vi "电源管理UI.vi"() -> ()   [LabVIEW 2016, in "PLC.lvlib"]
uses:
  PLC.lvlib
  <vilib>/Utility/miscctls.llb/LVPointTypeDef.ctl
  API/CodCr/CodCr.lvlib
  <vilib>/ptbypt/NI_PtbyPt.lvlib
panel:
  out "总氮空闲时间":dbl caption="空闲时间:"
  in  "总氮电源":bool
  out "CODCr空闲时间":dbl caption="空闲时间:"
  out "总磷空闲时间":dbl caption="空闲时间:"
  out "营养盐空闲时间":dbl caption="空闲时间:"
  out "CODMn空闲时间":dbl caption="空闲时间:"
  out "多参数空闲时间":dbl caption="空闲时间:"
  in  "CODCr电源":bool
  in  "总磷电源":bool
  in  "氨氮电源":bool
  in  "CODMn电源":bool
  in  "多参数电源":bool
  # "说明：\n系统模式处于维护模式时，仪器电源自动打开；\n系统模式处于常规模式/质控模式/应急模式下，周期启动时，仪器电源打开，仪器空闲超过3600秒自动断电；"
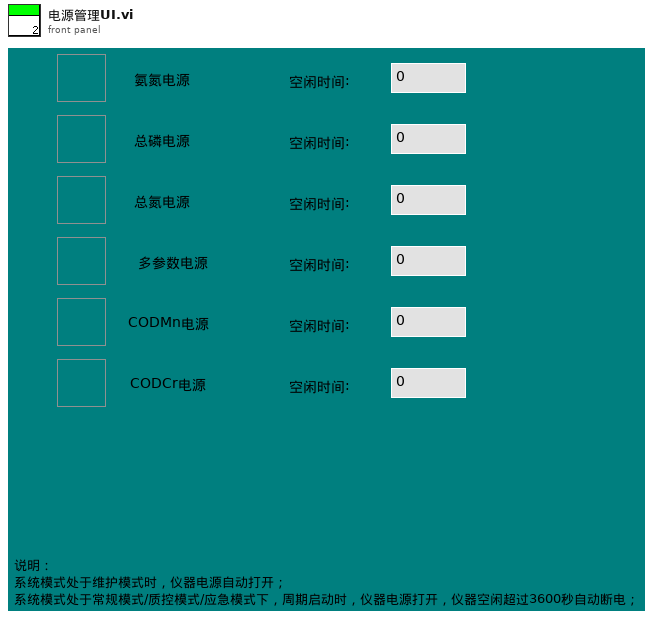
[diagram p1: front panel]
types:
  T1 = typedef "LVPointTypeDef.ctl" = cluster{"Horizontal":i16, "Vertical":i16}
  T2 = cluster{"测量量程":dbl, "测量精度":dbl, "测量间隔":dbl, "消解温度":dbl, "消解时长":dbl, "空白校准时间":timestamp, "曲线截距":dbl, "曲线斜率":dbl, "测量检出限":dbl, "测量信号值":dbl, "线性相关系数":dbl, "二次多项式系数":dbl, "标样校准时间":timestamp}
  T3 = cluster{"测量精度":u16, "消解温度":u16, "消解时长":u16, "量程下限":sgl, "量程上限":sgl, "曲线斜率K":sgl, "曲线斜率B":sgl, "标定日期":timestamp, "标液1浓度":sgl, "标液1测量过程值":sgl, "标液2浓度":sgl, "标液2测量过程值":sgl, "标液3浓度":sgl, "标液3测量过程值":sgl, "标液4浓度":sgl, "标液4测量过程值":sgl, "标液5浓度":sgl, "标液5测量过程值":sgl, "线性相关系数":sgl, "试剂余量":u32, "测量滴定值或吸光度":sgl, "空白校准时间":timestamp, "标样校准时间":timestamp, "检出限值":sgl, "校准系数":sgl, "设备系列号":string}
  T4 = enum16{"空闲", "水样测试", "标样核查", "零点核查", "跨度核查", "空白测试", "平行样测试", "加标回收", "空白校准", "标样校准", "初始化（清洗）"}
  T5 = cluster{"R0":i16, "R1":i16, "R2":i16, "R3":i16, "R4":i16, "R5":i16, "R6":i16, "R7":i16, "R8":i16, "R9":i16, "R10":i16, "R11":i16, "R12":i16, "R13":i16, "R14":i16, "R15":i16, "R16":i16, "R17":i16, "R18":i16, "R19":i16, "R20":i16, "R21":i16, "R22":i16, "R23":i16, "R24":i16, "R25":i16, "R26":i16, "R27":i16, "R28":i16, "R29":i16, "R30":i16, "R31":i16, "R32":i16, "R33":i16, "R34":i16, "R35":i16, "R36":i16, "R37":i16, "R38":i16, "R39":i16, "R40":i16, "R41":i16, "R42":i16, "R43":i16, "R44":i16, "R45":i16, "R46":i16, "R47":i16, "R48":i16, "R49":i16, "R50":i16, "R51":i16, "R52":i16, "R53":i16, "R54":i16, "R55":i16, "R56":i16}
  T6 = cluster{"系统时间":timestamp, "工作状态":enum16{"空闲", "水样测试", "标样核查", "零点核查", "跨度核查", "空白测试", "平行样测试", "加标回收", "空白校准", "标样校准", "初始化（清洗）"}, "测量模式":enum16{"待机", "连续模式", "周期模式", "定点模式", "受控模式", "手动模式"}, "告警代码":enum16{"无告警", "缺试剂告警", "缺水样告警", "缺蒸馏水告警", "缺标液告警", "仪表漏液告警", "标定异常告警", "超量程告警", "加热异常", "低试剂预警", "超上限告警", "超下限告警", "仪表内部其他异常", "滴定异常告警", "电极异常告警", "量程切换告警", "参数设置告警", "PH电极电位异常", "电导率电极异常", "浊度光度异常", "溶解氧电极异常", "溶解氧光强异常", "温度异常告警", "PH异常告警", "溶解氧异常告警", "电导率异常告警", "浊度异常告警", "叶绿素异常告警", "藻密度异常告警", "蓝绿藻异常告警", "ORP异常告警", "氨氮异常告警", "清洁刷异常告警", "SD卡异常告警", "蓝牙异常告警", "Wifi异常告警", "流程异常告警"}, "故障代码":enum16{"无故障", "电机故障", "温度故障", "通讯故障", "滴定故障"}, "日志代码":u16, "软件版本":u16, "F0":sgl, "F1":sgl, "F2":sgl, "F3":sgl, "T":sgl, "H":sgl, "id":u16, "flowid":u16, "量程":u16, "总磷控温温度1":sgl, "营养盐控温温度2":sgl, "ADC":sgl}
  T7 = cluster{"系统时间":timestamp, "工作状态":u16, "测量模式":u16, "告警代码":enum16{"无告警", "缺试剂告警", "缺水样告警", "缺蒸馏水告警", "缺标液告警", "仪表漏液告警", "标定异常告警", "超量程告警", "加热异常", "低试剂预警", "超上限告警", "超下限告警", "仪表内部其他异常", "滴定异常告警", "电极异常告警", "量程切换告警", "参数设置告警", "PH电极电位异常", "电导率电极异常", "浊度光度异常", "溶解氧电极异常", "溶解氧光强异常", "温度异常告警", "PH异常告警", "溶解氧异常告警", "电导率异常告警", "浊度异常告警", "叶绿素异常告警", "藻密度异常告警", "蓝绿藻异常告警", "ORP异常告警", "氨氮异常告警", "清洁刷异常告警", "SD卡异常告警", "蓝牙异常告警", "Wifi异常告警", "流程异常告警"}, "故障代码":enum16{"无故障", "电机故障", "温度故障", "通讯故障", "滴定故障"}, "日志代码":u16, "软件版本":string}
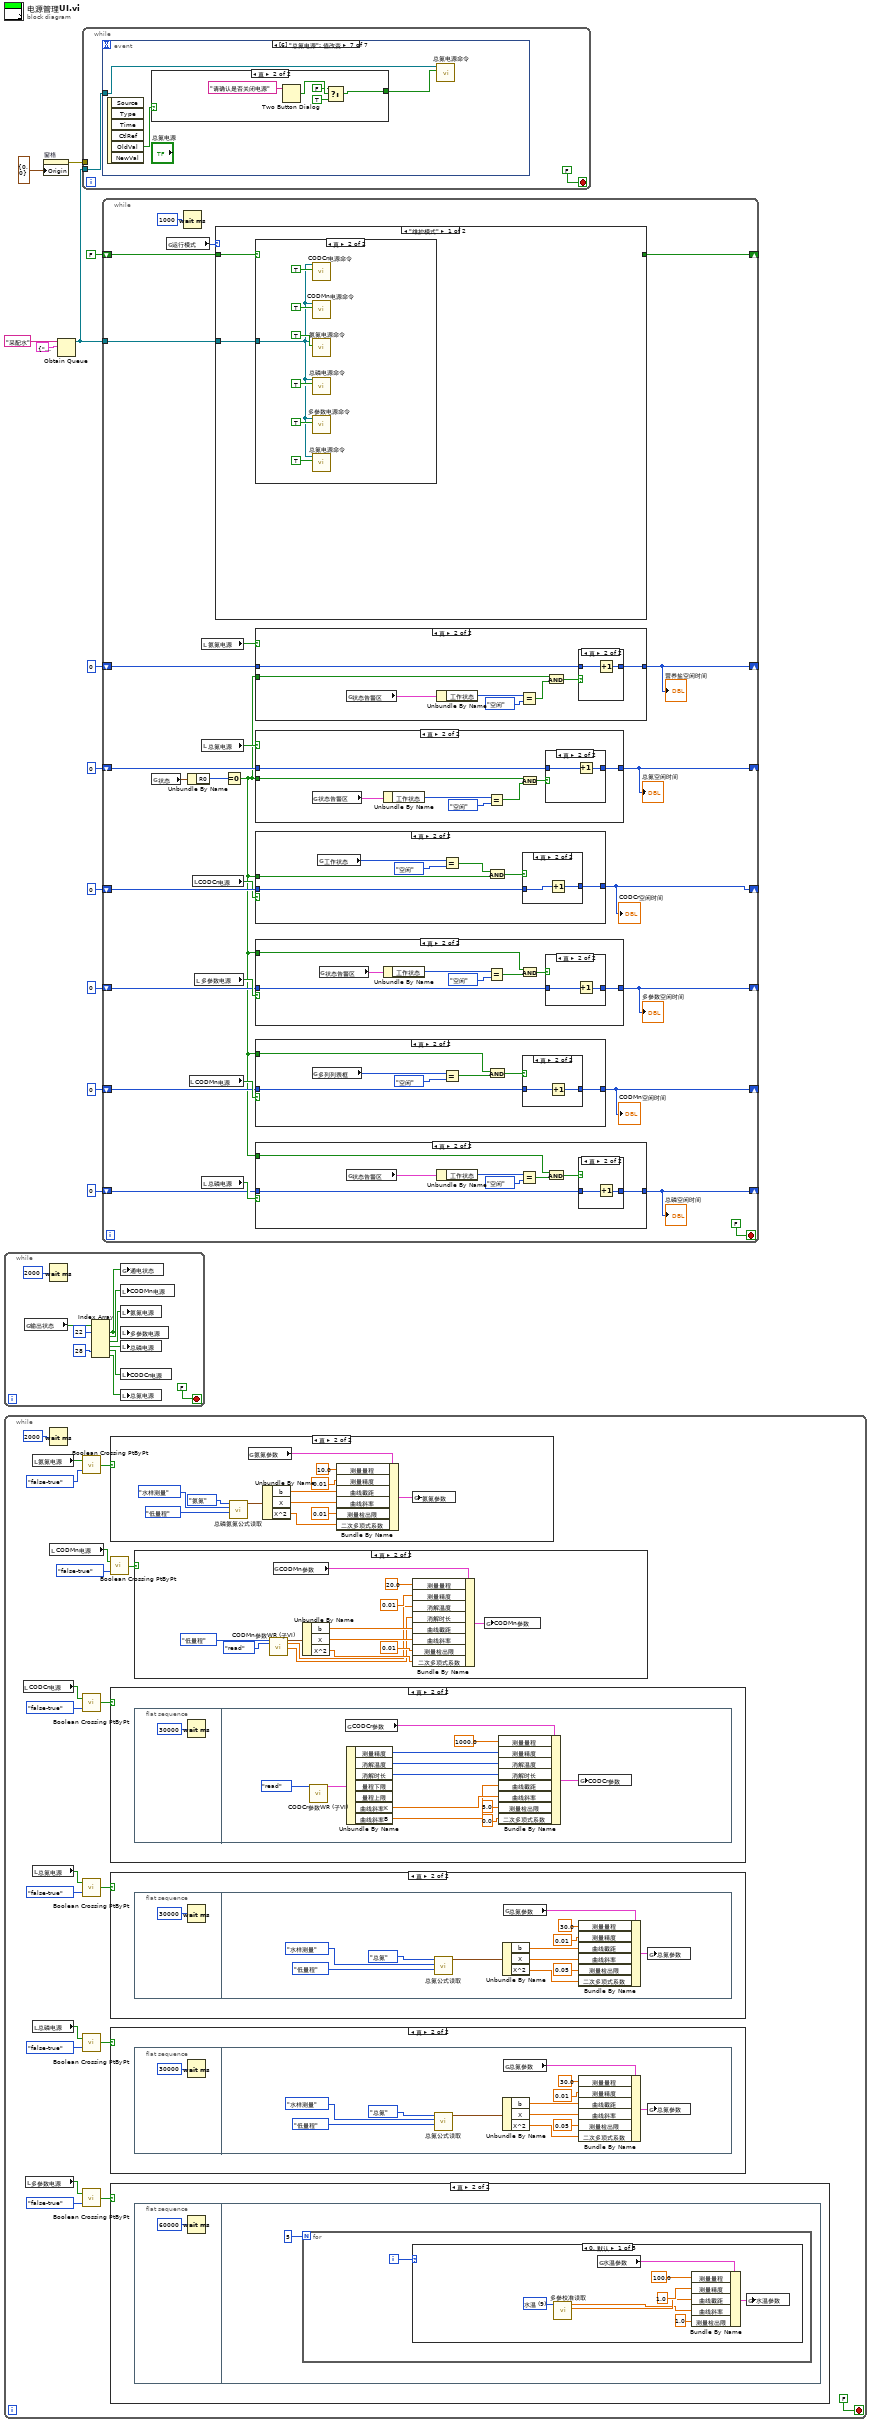
[diagram p0: block diagram]
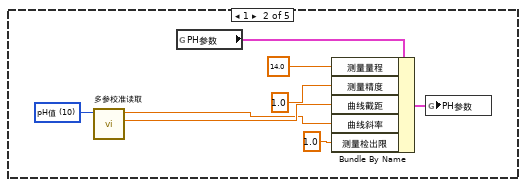
[diagram p8: hidden frame]
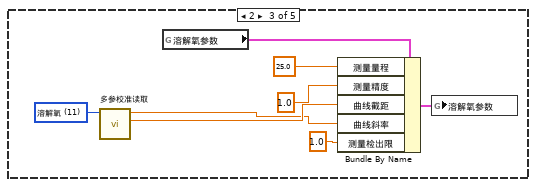
[diagram p9: hidden frame]
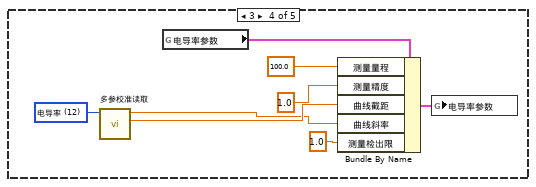
[diagram p10: hidden frame]
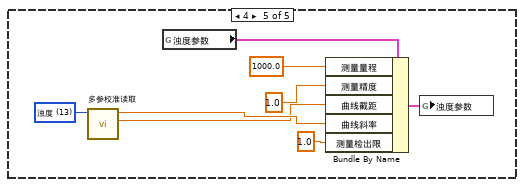
[diagram p11: hidden frame]
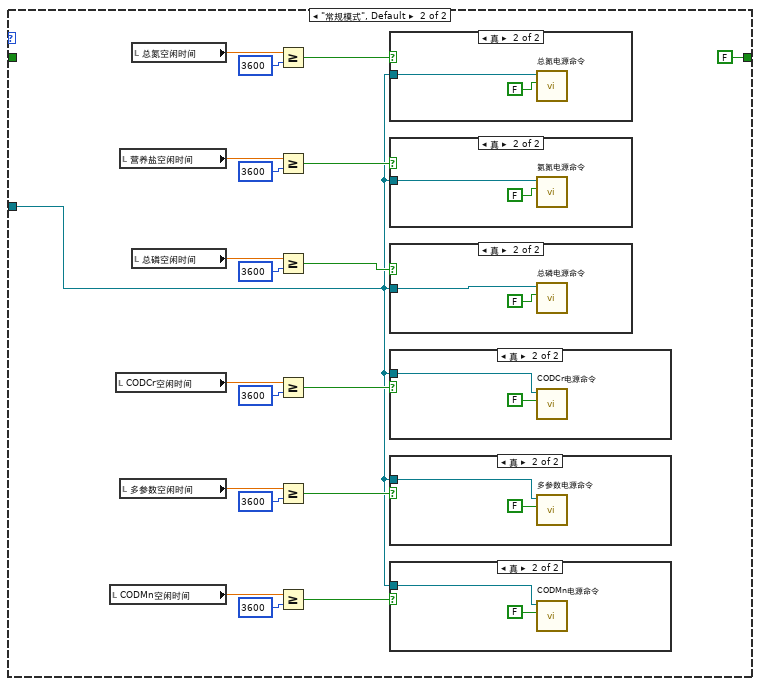
[diagram p15: hidden frame]
diagram:
  n1 = while {
    stop <- FALSE stop-if-true
    n2 = global read "采配水全局变量.vi" "输出状态"() -> (w21:bool[])
    n3 = Wait (ms)(milliseconds to wait=u32 2000 ("等待时间（毫秒）")) -> ()  [unwired: 1 out]
    n4 = Index Array(array=w21, index #1=22 ("索引"), index #5=28 ("索引")) -> (element #1=w16:bool, element #2=w19:bool, element #3=w18:bool, element #4=w17:bool, element #5=w14:bool, element #6=w13:bool)  [unwired: 4 in]
    n5 = global write "多参数全局变量.vi" "通电状态"(w16) -> ()
    n6 = local write "CODMn电源"(w19) -> ()
    n7 = local write "氨氮电源"(w18) -> ()
    n8 = local write "多参数电源"(w16) -> ()
    n9 = local write "总磷电源"(w17) -> ()
    n10 = local write "CODCr电源"(w14) -> ()
    n11 = local write "总氮电源"(w13) -> ()
  }
  n12 = while {
    stop <- FALSE stop-if-true
    n13 = local read "CODCr电源"() -> (w25:bool)
    n14 = local read "多参数电源"() -> (w41:bool)
    n15 = local read "氨氮电源"() -> (w34:bool)
    n16 = local read "总氮电源"() -> (w28:bool)
    n17 = local read "总磷电源"() -> (w31:bool)
    n18 = Wait (ms)(milliseconds to wait=u32 2000 ("等待时间（毫秒）")) -> ()  [unwired: 1 out]
    n19 = local read "CODMn电源"() -> (w37:bool)
    n20 = call <vilib>:"Boolean Crossing PtByPt.vi"("direction"=enum16{"either", "false-true", "true-false"}."false-true", "input"=w34) -> ("crossing"=w33:bool)  [unwired: 1 in]
    n21 = call <vilib>:"Boolean Crossing PtByPt.vi"("direction"=enum16{"either", "false-true", "true-false"}."false-true", "input"=w25) -> ("crossing"=w24:bool)  [unwired: 1 in]
    n22 = call <vilib>:"Boolean Crossing PtByPt.vi"("direction"=enum16{"either", "false-true", "true-false"}."false-true", "input"=w28) -> ("crossing"=w29:bool)  [unwired: 1 in]
    n23 = call <vilib>:"Boolean Crossing PtByPt.vi"("direction"=enum16{"either", "false-true", "true-false"}."false-true", "input"=w31) -> ("crossing"=w30:bool)  [unwired: 1 in]
    n24 = call <vilib>:"Boolean Crossing PtByPt.vi"("direction"=enum16{"either", "false-true", "true-false"}."false-true", "input"=w41) -> ("crossing"=w39:bool)  [unwired: 1 in]
    n25 = case shown="真" w33 {
      frame False {
      }
      frame True {
        n26 = call "总磷氨氮公式读取.vi"("量程"=enum16{"低量程", "高量程"}."低量程", "测量模式"=enum16{"水样测量", "空白核查", "跨度核查", "标样核查", "加标回收"}."水样测量", "测量参数"=enum16{"氨氮", "总磷"}."氨氮") -> ("公式"=w83:cluster{"X^2":dbl, "X":dbl, "b":dbl})  [unwired: 7 in, 1 out]
        n27 = global read "在线监测仪器仪表参数.vi" "氨氮参数"() -> (w87:T2)
        n28 = Unbundle By Name(w83) -> ("b"=w91:dbl, "X"=w92:dbl, "X^2"=w93:dbl)
        n29 = Bundle By Name(cluster=w87, "测量量程"=10.0, "测量精度"=0.01, "曲线截距"=w91, "曲线斜率"=w92, "测量检出限"=0.01, "二次多项式系数"=w93) -> (w88:T2)
        n30 = global write "在线监测仪器仪表参数.vi" "氨氮参数"(w88) -> ()
      }
    }
    n31 = call <vilib>:"Boolean Crossing PtByPt.vi"("direction"=enum16{"either", "false-true", "true-false"}."false-true", "input"=w37) -> ("crossing"=w36:bool)  [unwired: 1 in]
    n32 = case shown="真" w24 {
      frame False {
      }
      frame True {
        n33 = flat-sequence {
          frame #0 {
            n34 = Wait (ms)(milliseconds to wait=u32 30000 ("等待时间（毫秒）")) -> ()  [unwired: 1 out]
          }
          frame #1 {
            n35 = call "CODCr参数WR (子VI) .vi"("STEP"=enum16{"read", "writekb", "写入消解温度时间"}."read") -> ("关键参数区"=w46:T3)  [unwired: 17 in, 1 out]
            n36 = global read "在线监测仪器仪表参数.vi" "CODCr参数"() -> (w54:T2)
            n37 = Unbundle By Name(w46) -> ("测量精度"=w53:u16, "消解温度"=w47:u16, "消解时长"=w48:u16, "曲线斜率K"=w50:sgl, "曲线斜率B"=w49:sgl)  [unwired: 2 out]
            n38 = Bundle By Name(cluster=w54, "测量量程"=1000.0, "测量精度"=w53, "消解温度"=w47, "消解时长"=w48, "曲线截距"=w49, "曲线斜率"=w50, "测量检出限"=5.0, "二次多项式系数"=0.0) -> (w55:T2)
            n39 = global write "在线监测仪器仪表参数.vi" "CODCr参数"(w55) -> ()
          }
        }
      }
    }
    n40 = case shown="真" w29 {
      frame False {
      }
      frame True {
        n41 = flat-sequence {
          frame #0 {
            n42 = Wait (ms)(milliseconds to wait=u32 30000 ("等待时间（毫秒）")) -> ()  [unwired: 1 out]
          }
          frame #1 {
            n43 = call "总氮公式读取.vi"("量程"=enum16{"低量程", "高量程"}."低量程", "测量模式"=enum16{"水样测量", "空白核查", "跨度核查", "标样核查", "加标回收"}."水样测量", "测量参数"=enum16{"总磷", "总氮"}."总氮") -> ("公式"=w58:cluster{"X^2":dbl, "X":dbl, "b":dbl})  [unwired: 7 in, 1 out]
            n44 = Unbundle By Name(w58) -> ("b"=w67:dbl, "X"=w68:dbl, "X^2"=w69:dbl)
            n45 = global read "在线监测仪器仪表参数.vi" "总氮参数"() -> (w66:T2)
            n46 = Bundle By Name(cluster=w66, "测量量程"=30.0, "测量精度"=0.01, "曲线截距"=w67, "曲线斜率"=w68, "测量检出限"=0.05, "二次多项式系数"=w69) -> (w65:T2)
            n47 = global write "在线监测仪器仪表参数.vi" "总氮参数"(w65) -> ()
          }
        }
      }
    }
    n48 = case shown="真" w30 {
      frame False {
      }
      frame True {
        n49 = flat-sequence {
          frame #0 {
            n50 = Wait (ms)(milliseconds to wait=u32 30000 ("等待时间（毫秒）")) -> ()  [unwired: 1 out]
          }
          frame #1 {
            n51 = call "总氮公式读取.vi"("量程"=enum16{"低量程", "高量程"}."低量程", "测量模式"=enum16{"水样测量", "空白核查", "跨度核查", "标样核查", "加标回收"}."水样测量", "测量参数"=enum16{"总磷", "总氮"}."总氮") -> ("公式"=w71:cluster{"X^2":dbl, "X":dbl, "b":dbl})  [unwired: 7 in, 1 out]
            n52 = Unbundle By Name(w71) -> ("b"=w80:dbl, "X"=w81:dbl, "X^2"=w82:dbl)
            n53 = global read "在线监测仪器仪表参数.vi" "总氮参数"() -> (w79:T2)
            n54 = Bundle By Name(cluster=w79, "测量量程"=30.0, "测量精度"=0.01, "曲线截距"=w80, "曲线斜率"=w81, "测量检出限"=0.05, "二次多项式系数"=w82) -> (w78:T2)
            n55 = global write "在线监测仪器仪表参数.vi" "总氮参数"(w78) -> ()
          }
        }
      }
    }
    n56 = case shown="真" w39 {
      frame False {
      }
      frame True {
        n57 = flat-sequence {
          frame #0 {
            n58 = Wait (ms)(milliseconds to wait=u32 60000 ("等待时间（毫秒）")) -> ()  [unwired: 1 out]
          }
          frame #1 {
            n59 = for {
              N: 5 -> [_]
              i -> [w110]
              n60 = case shown="0, 默认" w110 {
                frame 0, Default {
                  w113 = u16 9 items=["氨氮"=3, "水温"=9, "pH值"=10, "溶解氧"=11, "电导率"=12, "浊度"=13, "叶绿素a"=14, "藻密度"=15, "蓝绿藻"=16, "氧化还原电位"=17, "溶解氧%"=18, "盐度"=19] ("站号")
                  n61 = call "多参校准读取.vi"("站号"=w113) -> ("B"=w112:dbl, "K"=w111:dbl)  [unwired: 8 in, 1 out]
                  n62 = global read "在线监测仪器仪表参数.vi" "水温参数"() -> (w115:T2)
                  n63 = Bundle By Name(cluster=w115, "测量量程"=100.0, "测量精度"=1.0, "曲线截距"=w112, "曲线斜率"=w111, "测量检出限"=1.0) -> (w116:T2)
                  n64 = global write "在线监测仪器仪表参数.vi" "水温参数"(w116) -> ()
                }
                frame 1 {
                  w121 = u16 10 items=["氨氮"=3, "水温"=9, "pH值"=10, "溶解氧"=11, "电导率"=12, "浊度"=13, "叶绿素a"=14, "藻密度"=15, "蓝绿藻"=16, "氧化还原电位"=17, "溶解氧%"=18, "盐度"=19] ("站号")
                  n65 = call "多参校准读取.vi"("站号"=w121) -> ("B"=w120:dbl, "K"=w119:dbl)  [unwired: 8 in, 1 out]
                  n66 = global read "在线监测仪器仪表参数.vi" "PH参数"() -> (w123:T2)
                  n67 = Bundle By Name(cluster=w123, "测量量程"=14.0, "测量精度"=1.0, "曲线截距"=w120, "曲线斜率"=w119, "测量检出限"=1.0) -> (w124:T2)
                  n68 = global write "在线监测仪器仪表参数.vi" "PH参数"(w124) -> ()
                }
                frame 2 {
                  w129 = u16 11 items=["氨氮"=3, "水温"=9, "pH值"=10, "溶解氧"=11, "电导率"=12, "浊度"=13, "叶绿素a"=14, "藻密度"=15, "蓝绿藻"=16, "氧化还原电位"=17, "溶解氧%"=18, "盐度"=19] ("站号")
                  n69 = call "多参校准读取.vi"("站号"=w129) -> ("B"=w128:dbl, "K"=w127:dbl)  [unwired: 8 in, 1 out]
                  n70 = global read "在线监测仪器仪表参数.vi" "溶解氧参数"() -> (w131:T2)
                  n71 = Bundle By Name(cluster=w131, "测量量程"=25.0, "测量精度"=1.0, "曲线截距"=w128, "曲线斜率"=w127, "测量检出限"=1.0) -> (w132:T2)
                  n72 = global write "在线监测仪器仪表参数.vi" "溶解氧参数"(w132) -> ()
                }
                frame 3 {
                  w137 = u16 12 items=["氨氮"=3, "水温"=9, "pH值"=10, "溶解氧"=11, "电导率"=12, "浊度"=13, "叶绿素a"=14, "藻密度"=15, "蓝绿藻"=16, "氧化还原电位"=17, "溶解氧%"=18, "盐度"=19] ("站号")
                  n73 = call "多参校准读取.vi"("站号"=w137) -> ("B"=w136:dbl, "K"=w135:dbl)  [unwired: 8 in, 1 out]
                  n74 = global read "在线监测仪器仪表参数.vi" "电导率参数"() -> (w139:T2)
                  n75 = Bundle By Name(cluster=w139, "测量量程"=100.0, "测量精度"=1.0, "曲线截距"=w136, "曲线斜率"=w135, "测量检出限"=1.0) -> (w140:T2)
                  n76 = global write "在线监测仪器仪表参数.vi" "电导率参数"(w140) -> ()
                }
                frame 4 {
                  w145 = u16 13 items=["氨氮"=3, "水温"=9, "pH值"=10, "溶解氧"=11, "电导率"=12, "浊度"=13, "叶绿素a"=14, "藻密度"=15, "蓝绿藻"=16, "氧化还原电位"=17, "溶解氧%"=18, "盐度"=19] ("站号")
                  n77 = call "多参校准读取.vi"("站号"=w145) -> ("B"=w143:dbl, "K"=w144:dbl)  [unwired: 8 in, 1 out]
                  n78 = global read "在线监测仪器仪表参数.vi" "浊度参数"() -> (w147:T2)
                  n79 = Bundle By Name(cluster=w147, "测量量程"=1000.0, "测量精度"=1.0, "曲线截距"=w143, "曲线斜率"=w144, "测量检出限"=1.0) -> (w148:T2)
                  n80 = global write "在线监测仪器仪表参数.vi" "浊度参数"(w148) -> ()
                }
              }
            }
          }
        }
      }
    }
    n81 = case shown="真" w36 {
      frame False {
      }
      frame True {
        n82 = call "CODMn参数WR (子VI).vi"("量程选择"=enum16{"低量程", "高量程"}."低量程", "STEP"=enum16{"read", "writekb", "写入消解温度时间"}."read") -> ("方程系数"=w99:cluster{"X^2":dbl, "X":dbl, "b":dbl}, "消解温度"=w98:dbl, "恒温时间"=w97:dbl)  [unwired: 14 in, 1 out]
        n83 = global read "在线监测仪器仪表参数.vi" "CODMn参数"() -> (w100:T2)
        n84 = Unbundle By Name(w99) -> ("b"=w105:dbl, "X"=w106:dbl, "X^2"=w107:dbl)
        n85 = Bundle By Name(cluster=w100, "测量量程"=20.0, "测量精度"=0.01, "消解温度"=w98, "消解时长"=w97, "曲线截距"=w105, "曲线斜率"=w106, "测量检出限"=0.01, "二次多项式系数"=w107) -> (w101:T2)
        n86 = global write "在线监测仪器仪表参数.vi" "CODMn参数"(w101) -> ()
      }
    }
  }
  n87 = property on="窗格" class="Pane"("Origin"=T1 {"Horizontal"=0, "Vertical"=0} ("原点")) -> (error out=w9:errorcluster)  [unwired: 2 in, 1 out]
  n88 = Obtain Queue(name (unnamed)="采配水" ("名称（未命名）"), element data type=cluster{"命令":string, "数据":variant} {"命令"="", "数据"=variant}) -> (queue out=w8:refnum<queue>)  [unwired: 3 in, 2 out]
  n89 = while {
    tunnel: w8 -> [w151]
    tunnel: w9 -> [_]
    stop <- FALSE stop-if-true
    n90 = event shown="[6] \"总氮电源\": 值改变" {
      selector: _ -> [_ _ _ _ _ _ _]
      dyn-events: _ -> [_ _ _ _ _ _ _]
      timeout: _ -> [_ _ _ _ _ _ _]
      tunnel: w151 -> [_ w155 w164 w173 w182 w191 w200]
      event Timeout {
        n91 = event-data() -> ()  [unwired: 1 in, 3 out]
      }
      event "多参数电源": Value Change {
        n92 = event-data() -> ("OldVal"=w154:bool)  [unwired: 1 in, 5 out]
        n93 = case shown="真" w154 {
          tunnel: [TRUE ("T button?") w157] -> w153
          frame False {
          }
          frame True {
            n94 = Two Button Dialog(message="请确认是否关闭电源" ("消息")) -> (T button?=w160:bool)  [unwired: 2 in]
            n95 = Select(t=FALSE, s=w160, f=TRUE ("T button?")) -> (s? t:f=w157:bool)
          }
        }
        n96 = call "多参数电源命令.vi"("通电/断电"=w153, "队列"=w155) -> ()  [unwired: 9 in, 1 out]
      }
      event "CODMn电源": Value Change {
        n97 = event-data() -> ("OldVal"=w163:bool)  [unwired: 1 in, 5 out]
        n98 = case shown="真" w163 {
          tunnel: [TRUE ("T button?") w166] -> w162
          frame False {
          }
          frame True {
            n99 = Two Button Dialog(message="请确认是否关闭电源" ("消息")) -> (T button?=w169:bool)  [unwired: 2 in]
            n100 = Select(t=FALSE, s=w169, f=TRUE ("T button?")) -> (s? t:f=w166:bool)
          }
        }
        n101 = call "CODMn电源命令.vi"("通电/断电"=w162, "队列"=w164) -> ()  [unwired: 9 in, 1 out]
      }
      event "氨氮电源": Value Change {
        n102 = event-data() -> ("OldVal"=w172:bool)  [unwired: 1 in, 5 out]
        n103 = case shown="真" w172 {
          tunnel: [TRUE ("T button?") w175] -> w171
          frame False {
          }
          frame True {
            n104 = Two Button Dialog(message="请确认是否关闭电源" ("消息")) -> (T button?=w178:bool)  [unwired: 2 in]
            n105 = Select(t=FALSE, s=w178, f=TRUE ("T button?")) -> (s? t:f=w175:bool)
          }
        }
        n106 = call "氨氮电源命令.vi"("通电/断电"=w171, "队列"=w173) -> ()  [unwired: 9 in, 1 out]
      }
      event "总磷电源": Value Change {
        n107 = event-data() -> ("OldVal"=w181:bool)  [unwired: 1 in, 5 out]
        n108 = case shown="真" w181 {
          tunnel: [TRUE ("T button?") w184] -> w180
          frame False {
          }
          frame True {
            n109 = Two Button Dialog(message="请确认是否关闭电源" ("消息")) -> (T button?=w187:bool)  [unwired: 2 in]
            n110 = Select(t=FALSE, s=w187, f=TRUE ("T button?")) -> (s? t:f=w184:bool)
          }
        }
        n111 = call "总磷电源命令.vi"("通电/断电"=w180, "队列"=w182) -> ()  [unwired: 9 in, 1 out]
      }
      event "CODCr电源": Value Change {
        n112 = event-data() -> ("OldVal"=w190:bool)  [unwired: 1 in, 5 out]
        n113 = case shown="真" w190 {
          tunnel: [TRUE ("T button?") w193] -> w189
          frame False {
          }
          frame True {
            n114 = Two Button Dialog(message="请确认是否关闭电源" ("消息")) -> (T button?=w196:bool)  [unwired: 2 in]
            n115 = Select(t=FALSE, s=w196, f=TRUE ("T button?")) -> (s? t:f=w193:bool)
          }
        }
        n116 = call "CODCr电源命令.vi"("通电/断电"=w189, "队列"=w191) -> ()  [unwired: 9 in, 1 out]
      }
      event "总氮电源": Value Change {
        n117 = event-data() -> ("OldVal"=w198:bool)  [unwired: 1 in, 5 out]
        n118 = case shown="真" w198 {
          tunnel: [TRUE ("T button?") w202] -> w199
          frame False {
          }
          frame True {
            n119 = Two Button Dialog(message="请确认是否关闭电源" ("消息")) -> (T button?=w205:bool)  [unwired: 2 in]
            n120 = Select(t=FALSE, s=w205, f=TRUE ("T button?")) -> (s? t:f=w202:bool)
          }
        }
        n121 = call "总氮电源命令.vi"("通电/断电"=w199, "队列"=w200) -> ()  [unwired: 9 in, 1 out]
      }
    }
  }
  n122 = while {
    tunnel: w8 -> [w216]
    shift-right: [w217] -> _
    shift-left: u32 0 ("等待时间（毫秒）") -> [w230]
    shift-right: [w221] -> _
    shift-left: u32 0 ("等待时间（毫秒）") -> [w228]
    shift-right: [w219] -> _
    shift-left: u32 0 ("等待时间（毫秒）") -> [w224]
    shift-right: [w220] -> _
    shift-left: u32 0 ("等待时间（毫秒）") -> [w225]
    shift-right: [w218] -> _
    shift-left: u32 0 ("等待时间（毫秒）") -> [w223]
    shift-right: [w213] -> _
    shift-left: FALSE -> [w214]
    shift-right: [w207] -> _
    shift-left: u32 0 ("等待时间（毫秒）") -> [w209]
    stop <- FALSE stop-if-true
    n123 = global read "采配水全局变量.vi" "状态"() -> (w212:T5)
    n124 = global read "系统变量.vi" "运行模式"() -> (w215:enum16{"维护模式", "常规模式", "应急模式", "质控模式"})
    n125 = Wait (ms)(milliseconds to wait=u32 1000 ("等待时间（毫秒）")) -> ()  [unwired: 1 out]
    n126 = Unbundle By Name(w212) -> ("R0"=w211:i16)
    n127 = local read "CODMn电源"() -> (w229:bool)
    n128 = local read "CODCr电源"() -> (w222:bool)
    n129 = local read "多参数电源"() -> (w226:bool)
    n130 = local read "氨氮电源"() -> (w231:bool)
    n131 = local read "总氮电源"() -> (w210:bool)
    n132 = local read "总磷电源"() -> (w227:bool)
    n133 = case shown="\"维护模式\"" w215 {
      tunnel: w216 -> [w245 w253]
      tunnel: w214 -> [w244 _]
      tunnel: [_ FALSE] -> w213
      frame "维护模式" {
        n134 = case shown="真" w244 {
          tunnel: w245 -> [_ w247]
          frame False {
          }
          frame True {
            n135 = call "CODCr电源命令.vi"("通电/断电"=TRUE, "队列"=w247) -> ()  [unwired: 9 in, 1 out]
            n136 = call "CODMn电源命令.vi"("通电/断电"=TRUE, "队列"=w247) -> ()  [unwired: 9 in, 1 out]
            n137 = call "氨氮电源命令.vi"("通电/断电"=TRUE, "队列"=w247) -> ()  [unwired: 9 in, 1 out]
            n138 = call "总磷电源命令.vi"("通电/断电"=TRUE, "队列"=w247) -> ()  [unwired: 9 in, 1 out]
            n139 = call "多参数电源命令.vi"("通电/断电"=TRUE, "队列"=w247) -> ()  [unwired: 9 in, 1 out]
            n140 = call "总氮电源命令.vi"("通电/断电"=TRUE, "队列"=w247) -> ()  [unwired: 9 in, 1 out]
          }
        }
      }
      frame "常规模式", Default {
        n141 = local read "CODMn空闲时间"() -> (w261:dbl)
        n142 = local read "CODCr空闲时间"() -> (w268:dbl)
        n143 = local read "营养盐空闲时间"() -> (w264:dbl)
        n144 = local read "多参数空闲时间"() -> (w267:dbl)
        n145 = local read "总氮空闲时间"() -> (w256:dbl)
        n146 = local read "总磷空闲时间"() -> (w258:dbl)
        n147 = Greater Or Equal?(x=w256, y=u32 3600) -> (x >= y?=w254:bool)
        n148 = Greater Or Equal?(x=w264, y=u32 3600) -> (x >= y?=w266:bool)
        n149 = Greater Or Equal?(x=w258, y=u32 3600) -> (x >= y?=w260:bool)
        n150 = Greater Or Equal?(x=w268, y=u32 3600) -> (x >= y?=w270:bool)
        n151 = Greater Or Equal?(x=w267, y=u32 3600) -> (x >= y?=w272:bool)
        n152 = Greater Or Equal?(x=w261, y=u32 3600) -> (x >= y?=w263:bool)
        n153 = case shown="真" w254 {
          tunnel: w253 -> [_ w274]
          frame False {
          }
          frame True {
            n154 = call "总氮电源命令.vi"("通电/断电"=FALSE, "队列"=w274) -> ()  [unwired: 9 in, 1 out]
          }
        }
        n155 = case shown="真" w266 {
          tunnel: w253 -> [_ w280]
          frame False {
          }
          frame True {
            n156 = call "氨氮电源命令.vi"("通电/断电"=FALSE, "队列"=w280) -> ()  [unwired: 9 in, 1 out]
          }
        }
        n157 = case shown="真" w260 {
          tunnel: w253 -> [_ w276]
          frame False {
          }
          frame True {
            n158 = call "总磷电源命令.vi"("通电/断电"=FALSE, "队列"=w276) -> ()  [unwired: 9 in, 1 out]
          }
        }
        n159 = case shown="真" w270 {
          tunnel: w253 -> [_ w282]
          frame False {
          }
          frame True {
            n160 = call "CODCr电源命令.vi"("通电/断电"=FALSE, "队列"=w282) -> ()  [unwired: 9 in, 1 out]
          }
        }
        n161 = case shown="真" w272 {
          tunnel: w253 -> [_ w284]
          frame False {
          }
          frame True {
            n162 = call "多参数电源命令.vi"("通电/断电"=FALSE, "队列"=w284) -> ()  [unwired: 9 in, 1 out]
          }
        }
        n163 = case shown="真" w263 {
          tunnel: w253 -> [_ w278]
          frame False {
          }
          frame True {
            n164 = call "CODMn电源命令.vi"("通电/断电"=FALSE, "队列"=w278) -> ()  [unwired: 9 in, 1 out]
          }
        }
      }
    }
    n165 = Equal To 0?(x=w211) -> (x = 0?=w208:bool)
    n166 = case shown="真" w231 {
      tunnel: w230 -> [_ w330]
      tunnel: [_ w326] -> w217
      tunnel: w208 -> [_ w323]
      frame False {
      }
      frame True {
        n167 = global read "VAR总磷氨氮全局变量.vi" "状态告警区"() -> (w325:T6)
        n168 = Unbundle By Name(w325) -> ("工作状态"=w329:T4)
        n169 = Equal?(x=w329, y=T4."空闲" ("工作状态")) -> (x = y?=w327:bool)
        n170 = And(x=w323, y=w327) -> (x .and. y?=w324:bool)
        n171 = case shown="真" w324 {
          tunnel: w330 -> [_ w332]
          tunnel: [_ w331] -> w326
          frame False {
          }
          frame True {
            n172 = Increment(x=w332) -> (x+1=w331:u32)
          }
        }
      }
    }
    "营养盐空闲时间" <- w217
    n173 = case shown="真" w210 {
      tunnel: w209 -> [_ w241]
      tunnel: [_ w238] -> w207
      tunnel: w208 -> [_ w235]
      frame False {
      }
      frame True {
        n174 = global read "VAR总氮全局变量.vi" "状态告警区"() -> (w234:T6)
        n175 = Unbundle By Name(w234) -> ("工作状态"=w237:T4)
        n176 = Equal?(x=w237, y=T4."空闲" ("工作状态")) -> (x = y?=w239:bool)
        n177 = And(x=w235, y=w239) -> (x .and. y?=w236:bool)
        n178 = case shown="真" w236 {
          tunnel: w241 -> [_ w243]
          tunnel: [_ w242] -> w238
          frame False {
          }
          frame True {
            n179 = Increment(x=w243) -> (x+1=w242:u32)
          }
        }
      }
    }
    "总氮空闲时间" <- w207
    n180 = case shown="真" w222 {
      tunnel: w223 -> [_ w291]
      tunnel: [_ w288] -> w218
      tunnel: w208 -> [_ w285]
      frame False {
      }
      frame True {
        n181 = global read "CODcr全局变量.vi" "工作状态"() -> (w287:T4)
        n182 = Equal?(x=w287, y=T4."空闲" ("工作状态")) -> (x = y?=w289:bool)
        n183 = And(x=w289, y=w285) -> (x .and. y?=w286:bool)
        n184 = case shown="真" w286 {
          tunnel: w291 -> [_ w293]
          tunnel: [_ w292] -> w288
          frame False {
          }
          frame True {
            n185 = Increment(x=w293) -> (x+1=w292:u32)
          }
        }
      }
    }
    "CODCr空闲时间" <- w218
    n186 = case shown="真" w226 {
      tunnel: w224 -> [_ w301]
      tunnel: [_ w298] -> w219
      tunnel: w208 -> [_ w294]
      frame False {
      }
      frame True {
        n187 = global read "多参数全局变量.vi" "状态告警区"() -> (w297:T7)
        n188 = Unbundle By Name(w297) -> ("工作状态"=w296:u16)
        n189 = Equal?(x=w296, y=T4."空闲" ("工作状态")) -> (x = y?=w299:bool)
        n190 = And(x=w294, y=w299) -> (x .and. y?=w295:bool)
        n191 = case shown="真" w295 {
          tunnel: w301 -> [_ w303]
          tunnel: [_ w302] -> w298
          frame False {
          }
          frame True {
            n192 = Increment(x=w303) -> (x+1=w302:u32)
          }
        }
      }
    }
    "多参数空闲时间" <- w219
    n193 = case shown="真" w229 {
      tunnel: w228 -> [_ w320]
      tunnel: [_ w317] -> w221
      tunnel: w208 -> [_ w314]
      frame False {
      }
      frame True {
        n194 = global read "运行时序全局变量.vi" "多列列表框"() -> (w316:i32)
        n195 = Equal?(x=w316, y=T4."空闲" ("工作状态")) -> (x = y?=w318:bool)
        n196 = And(x=w314, y=w318) -> (x .and. y?=w315:bool)
        n197 = case shown="真" w315 {
          tunnel: w320 -> [_ w322]
          tunnel: [_ w321] -> w317
          frame False {
          }
          frame True {
            n198 = Increment(x=w322) -> (x+1=w321:u32)
          }
        }
      }
    }
    "CODMn空闲时间" <- w221
    n199 = case shown="真" w227 {
      tunnel: w225 -> [_ w311]
      tunnel: [_ w308] -> w220
      tunnel: w208 -> [_ w304]
      frame False {
      }
      frame True {
        n200 = global read "VAR总磷氨氮全局变量.vi" "状态告警区"() -> (w307:T6)
        n201 = Unbundle By Name(w307) -> ("工作状态"=w306:T4)
        n202 = Equal?(x=w306, y=T4."空闲" ("工作状态")) -> (x = y?=w309:bool)
        n203 = And(x=w304, y=w309) -> (x .and. y?=w305:bool)
        n204 = case shown="真" w305 {
          tunnel: w311 -> [_ w313]
          tunnel: [_ w312] -> w308
          frame False {
          }
          frame True {
            n205 = Increment(x=w313) -> (x+1=w312:u32)
          }
        }
      }
    }
    "总磷空闲时间" <- w220
  }
